vi "CFunc.lua.vi"(0 "L":u64, 1 "Path":path) -> ()   [LabVIEW 2014]
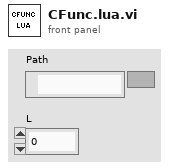
[diagram p1: front panel]
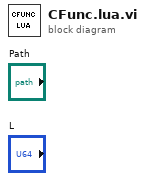
[diagram p0: block diagram]
diagram:
